vi "createEvents.vi"(8 "error in (no error)":errorcluster, 11 "MonoPubSubData in":refnum<class "MonoPubSubData.lvclass">) -> (0 "error out":errorcluster, 3 "MonoPubSubData out":refnum<class "MonoPubSubData.lvclass">)   [LabVIEW 2020, in "MonoPubSubData.lvclass"]
uses:
  MonoPubSubData.lvclass
  Typedefs/slit.ctl
  Typedefs/SlitType.ctl
  Typedefs/slitWidth.ctl
  Typedefs/GratingType.ctl
  Typedefs/wavelength.ctl
  Typedefs/DeviceStatus.ctl
  Typedefs/AckType.ctl
  MonoPubSubData.lvclass/MonoPubSubData.ctl
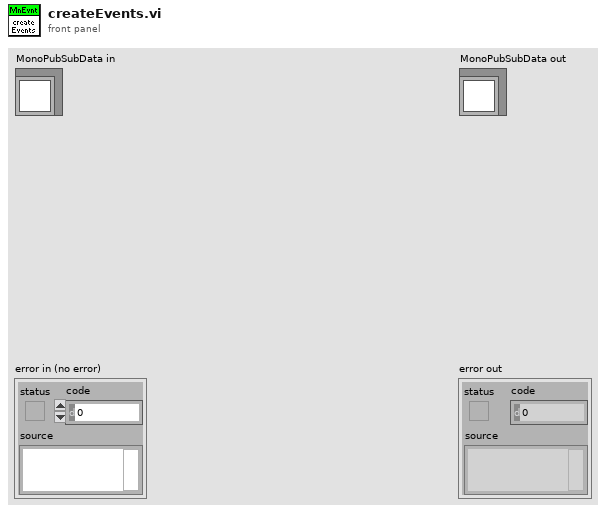
[diagram p1: front panel]
types:
  T1 = typedef "wavelength.ctl" = dbl
  T2 = typedef "slitWidth.ctl" = dbl
  T3 = typedef "GratingType.ctl" = enum16{"Blue", "Red", "Mirror"}
  T4 = cluster{"wavelength":T1, "frontExitSlitWidth":T2, "fronEntranceSlitWidth":T2, "GratingType":T3}
  T5 = typedef "AckType.ctl" = enum16{"OK", "OutOfRange", "Unknown", "Busy", "Rejected"}
  T6 = typedef "SlitType.ctl" = enum16{"Front Entrance", "Side Entrance", "Front Exit", "Side Exit", "First Intermediate", "Second Intermediate"}
  T7 = typedef "slit.ctl" = cluster{"SlitType":T6, "Width":T2}
  T8 = typedef "DeviceStatus.ctl" = enum16{"SettingUp", "Ready", "Offline", "Fault"}
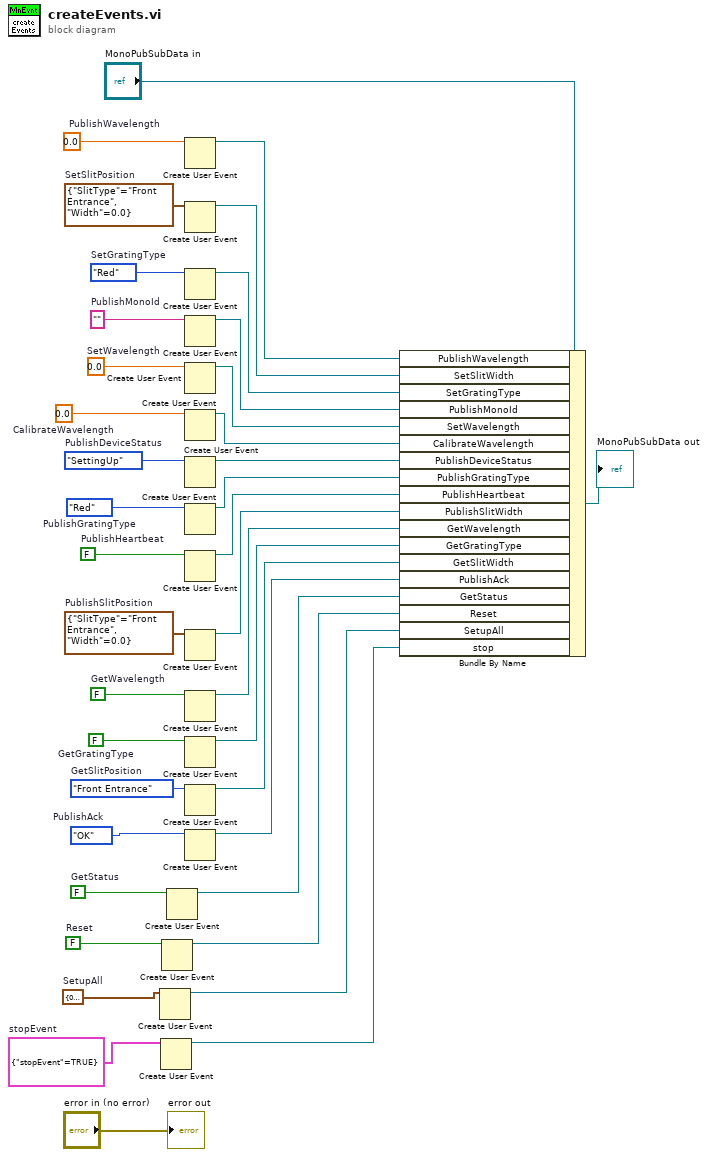
[diagram p0: block diagram]
diagram:
  w2 = cluster{"stopEvent":bool} {"stopEvent"=TRUE}  # stopEvent
  w4 = T4 {"wavelength"=0.0, "frontExitSlitWidth"=0.0, "fronEntranceSlitWidth"=0.0, "GratingType"=enum."Blue"}  # SetupAll
  w6 = FALSE  # Reset
  w8 = FALSE  # GetStatus
  w10 = AckType."OK"  # PublishAck
  w12 = SlitType."Front Entrance"  # GetSlitPosition
  w15 = FALSE  # GetWavelength
  w16 = FALSE  # GetGratingType
  w29 = T1 0.0  # PublishWavelength
  w30 = ""  # PublishMonoId
  w31 = FALSE  # PublishHeartbeat
  w32 = T7 {"SlitType"=enum."Front Entrance", "Width"=0.0}  # PublishSlitPosition
  w33 = GratingType."Red"  # PublishGratingType
  w34 = DeviceStatus."SettingUp"  # PublishDeviceStatus
  w35 = T1 0.0  # CalibrateWavelength
  w36 = T1 0.0  # SetWavelength
  w37 = GratingType."Red"  # SetGratingType
  w38 = T7 {"SlitType"=enum."Front Entrance", "Width"=0.0}  # SetSlitPosition
  n1 = Create User Event(user event datatype=w4) -> (user event=w3:refnum<user-event>)  [unwired: 1 in, 1 out]
  n2 = Create User Event(user event datatype=w2) -> (user event=w1:refnum<user-event>)  [unwired: 1 in, 1 out]
  n3 = Create User Event(user event datatype=w6) -> (user event=w5:refnum<user-event>)  [unwired: 1 in, 1 out]
  n4 = Create User Event(user event datatype=w8) -> (user event=w7:refnum<user-event>)  [unwired: 1 in, 1 out]
  n5 = Create User Event(user event datatype=w29) -> (user event=w23:refnum<user-event>)  [unwired: 1 in, 1 out]
  n6 = Create User Event(user event datatype=w38) -> (user event=w19:refnum<user-event>)  [unwired: 1 in, 1 out]
  n7 = Create User Event(user event datatype=w37) -> (user event=w18:refnum<user-event>)  [unwired: 1 in, 1 out]
  n8 = Create User Event(user event datatype=w30) -> (user event=w24:refnum<user-event>)  [unwired: 1 in, 1 out]
  n9 = Create User Event(user event datatype=w36) -> (user event=w21:refnum<user-event>)  [unwired: 1 in, 1 out]
  n10 = Create User Event(user event datatype=w35) -> (user event=w20:refnum<user-event>)  [unwired: 1 in, 1 out]
  n11 = Create User Event(user event datatype=w34) -> (user event=w22:refnum<user-event>)  [unwired: 1 in, 1 out]
  n12 = Create User Event(user event datatype=w33) -> (user event=w17:refnum<user-event>)  [unwired: 1 in, 1 out]
  n13 = Create User Event(user event datatype=w31) -> (user event=w25:refnum<user-event>)  [unwired: 1 in, 1 out]
  n14 = Create User Event(user event datatype=w32) -> (user event=w26:refnum<user-event>)  [unwired: 1 in, 1 out]
  n15 = Create User Event(user event datatype=w15) -> (user event=w14:refnum<user-event>)  [unwired: 1 in, 1 out]
  n16 = Create User Event(user event datatype=w16) -> (user event=w13:refnum<user-event>)  [unwired: 1 in, 1 out]
  n17 = Create User Event(user event datatype=w12) -> (user event=w11:refnum<user-event>)  [unwired: 1 in, 1 out]
  n18 = Create User Event(user event datatype=w10) -> (user event=w9:refnum<user-event>)  [unwired: 1 in, 1 out]
  n19 = Bundle By Name(cluster="MonoPubSubData in", "PublishWavelength"=w23, "SetSlitWidth"=w19, "SetGratingType"=w18, "PublishMonoId"=w24, "SetWavelength"=w21, "CalibrateWavelength"=w20, "PublishDeviceStatus"=w22, "PublishGratingType"=w17, "PublishHeartbeat"=w25, "PublishSlitWidth"=w26, "GetWavelength"=w14, "GetGratingType"=w13, "GetSlitWidth"=w11, "PublishAck"=w9, "GetStatus"=w7, "Reset"=w5, "SetupAll"=w3, "stop"=w1) -> (→"MonoPubSubData out":refnum<class "MonoPubSubData.lvclass">)
  "error out" <- "error in (no error)"
